vi "get_RegistrationArray.vi"(3 "error in (no error)":errorcluster, 5 "HGF_SVMonitorVisitor_getReg in":refnum<class "HGF_SVMonitorVisitor_getReg.lvclass">) -> (0 "error out":errorcluster, 1 "Registration Array":T1(array[cluster]), 2 "HGF_SVMonitorVisitor_getReg out":refnum<class "HGF_SVMonitorVisitor_getReg.lvclass">)   [LabVIEW 2012, in "HGF_SV.lvlib" / "HGF_SVMonitorVisitor_getReg.lvclass"]
uses:
  HGF_SVMonitorVisitor_getReg.lvclass
  HGF_BaseClasses/HGF_NetworkVisitor/HGF_NetworkVisitor.lvclass
  HGF_BaseClasses/HGF_TriggeredEvent/HGF_TriggeredEvent.lvclass
  HGF_SVMonitorVisitor_getReg.lvclass/HGF_SVMonitorVisitor_getReg.ctl
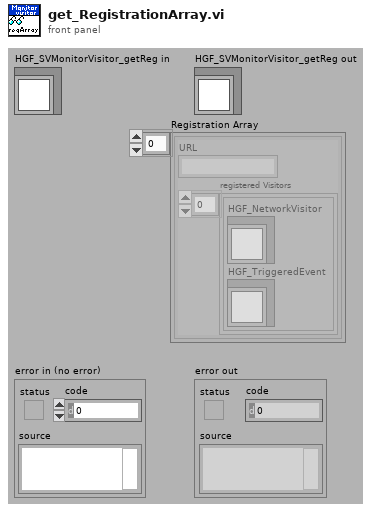
[diagram p1: front panel]
types:
  T1 = cluster{"URL":string, "registered Visitors":cluster{"HGF_NetworkVisitor":refnum<class "HGF_NetworkVisitor.lvclass">, "HGF_TriggeredEvent":refnum<class "HGF_TriggeredEvent.lvclass">}[]}[]
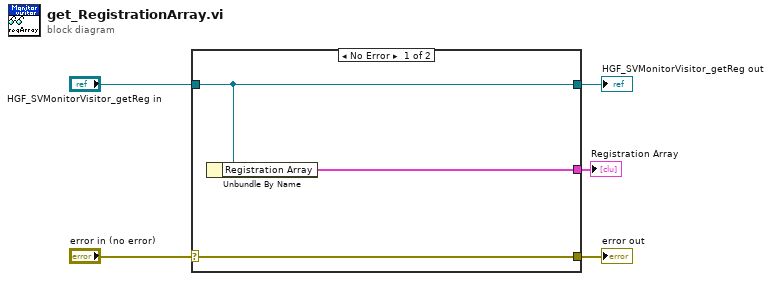
[diagram p0: block diagram]
diagram:
  n1 = case shown="No Error" "error in (no error)" {
    selector: "error in (no error)" -> [w8 w9]
    tunnel: [w8 w9] -> w4
    tunnel: [w7 w10] -> w2
    tunnel: "HGF_SVMonitorVisitor_getReg in" -> [w7 w10]
    tunnel: [w6 _] -> w1
    frame No Error {
      n2 = Unbundle By Name(w7) -> ("Registration Array"=w6:T1)
    }
    frame Error {
    }
  }
  "error out" <- w4
  "HGF_SVMonitorVisitor_getReg out" <- w2
  "Registration Array" <- w1
